vi "Launcher.vi"() -> ()   [LabVIEW 2023]
uses:
  Internal Communication/Controls/State FGV.ctl
  <vilib>/FPGAPlugInAG/Dynamic/niLvFpga_Close_Dynamic.vi
  <vilib>/rvi/interface/nirviCloseFPGA/nirviCloseFPGA.xnode
  Heart/Heart.lvlib
  Internal Communication/Internal Communication.lvlib
  FPGA/FPGA.lvlib
  Error Handling/Error Handling.lvlib
  Decoder/Decoder.lvlib
  Encoder/Encoder.lvlib
panel:
  in  "error in (no error)":errorcluster
  out "error out":errorcluster
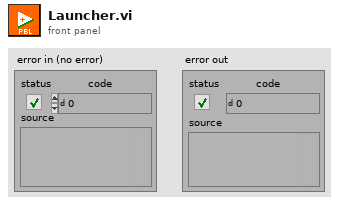
[diagram p1: front panel]
types:
  T1 = typedef "Internal Communication.lvlib/State FGV.ctl" = enum16{"Create Queues", "Get Queues", "Destroy Queues"}
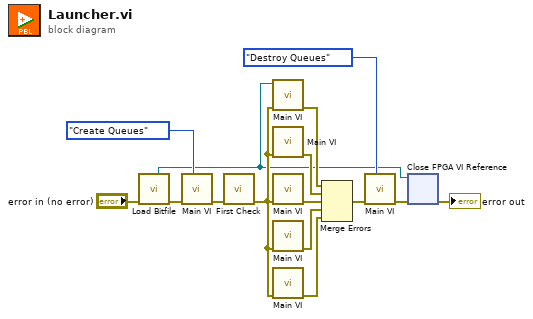
[diagram p0: block diagram]
diagram:
  n1 = call "Load Bitfile.vi"("error in"="error in (no error)") -> ("error out"=w4:errorcluster, "FPGA VI Reference Out"=w1:refnum<k20>)  [unwired: 9 in]
  n2 = call "Main VI.vi"("Enum"=State_FGV."Create Queues", "error in (no error)"=w4) -> ("error out"=w14:errorcluster)  [unwired: 8 in, 1 out]
  n3 = call "First Check.vi"("error in (no error)"=w14) -> ("error out"=w7:errorcluster)  [unwired: 10 in]
  n4 = call "Main VI.vi"("error in (no error)"=w7, "FPGA VI Reference In"=w1) -> ("error out"=w10:errorcluster)  [unwired: 9 in]
  n5 = call "Main VI.vi"("error in"=w7) -> ("error out"=w13:errorcluster)  [unwired: 10 in]
  n6 = call "Main VI.vi"("error in (no error)"=w7) -> ("error out"=w12:errorcluster)  [unwired: 9 in, 1 out]
  n7 = call "Main VI.vi"("error in"=w7) -> ("error out"=w11:errorcluster)  [unwired: 10 in]
  n8 = call "Main VI.vi"("error in (no error)"=w7) -> ("error out"=w6:errorcluster)  [unwired: 10 in]
  n9 = Merge Errors(w10, w13, w12, w11, w6) -> (w9:errorcluster)
  n10 = call "Main VI.vi"("Enum"=State_FGV."Destroy Queues", "error in (no error)"=w9) -> ("error out"=w3:errorcluster)  [unwired: 8 in, 1 out]
  n11 = xnode "Close FPGA VI Reference"("FPGA VI Reference In"=w1, "error in"=w3) -> ("error out"=→"error out":errorcluster)
